vi "PH_TKTDS-30xx.Revision.vi"(0 "i ref in":refnum<vi>, 5 "error IO":errorcluster) -> (14 "i ref out":refnum<vi>, 19 "error out":errorcluster)   [LabVIEW 2014, in "PH_TKTDS-30xx.lvlib"]
doc: "If the connection is established, this VI queries the instrumnent driver revision, the instrument firmware revision, and errors which are written to own attributes."
uses:
  PH_TKTDS-30xx.lvlib
  instr.lib/TKDS3032-PHELIX/tktds3032-PHELIX - Driver np.lvlib
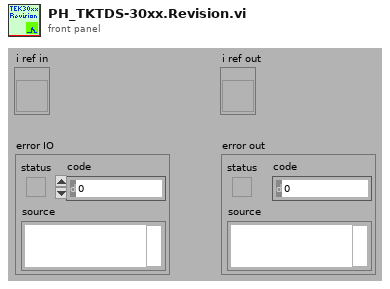
[diagram p1: front panel]
types:
  T1 = typedef "PH_TKTDS-30xx.lvlib/PH_TKTDS-30xx.i attribute.ctl" = cluster{"Default VISA Resource":string, "VISA Resource Name":refnum<visa-resource-name>, "Revision":cluster{"Instrument Driver":string, "Instrument Firmware":string}, "Selftest":cluster{"Result":u32, "Message":string}, "Channels":T2[], "Trigger Configuration":T3, "Acquisition Configuration":T4, "Fetched Waveforms":T5[], "GUI Refs":T6, "GUI Refs Channels":refnum<vi>[], "State":T7, "Error Message":string, "Allow Prdc Loop?":bool}
  T2 = typedef "PH_TKTDS-30xx.lvlib/PH_TKTDS-30xx.Channel Config.ctl" = cluster{"Channel Name":string, "Input Impedance":string, "Max Input Frequency":string, "Vertical Coupling":i32, "Channel Enabled":bool, "Probe Attenuation":dbl, "Vertical Range":dbl, "Vertical Offset":dbl}
  T3 = typedef "PH_TKTDS-30xx.lvlib/PH_TKTDS-30xx.Trigger Config.ctl" = cluster{"Source":string, "Slope":i32, "Level [V]":dbl}
  T4 = typedef "PH_TKTDS-30xx.lvlib/PH_TKTDS-30xx.Acquisition Config.ctl" = cluster{"Time base":dbl, "Record Length":u16, "Start Time":dbl, "Type":i32, "Continuous":bool}
  T5 = typedef "PH_TKTDS-30xx.lvlib/PH_TKTDS-30xx.fetched Waveform.ctl" = cluster{"Source":string, "Actual Points":u32, "Initial X":dbl, "X Increment":dbl, "Waveform Array":dbl[]}
  T6 = typedef "PH_TKTDS-30xx.lvlib/PH_TKTDS-30xx.GUI Refs.ctl" = cluster{"Trigger":refnum<vi>, "Acquisition":refnum<vi>, "Graph":refnum<vi>, "State":refnum<vi>, "Delete":refnum<vi>, "Channel to be positioned":refnum<vi>, "Postion":refnum<vi>, "Display Intensity":refnum<vi>, "VISA Resource":refnum<vi>}
  T7 = typedef "PH_StatusHandler.lvlib/PH_StatusHandler.Status.ctl" = i16
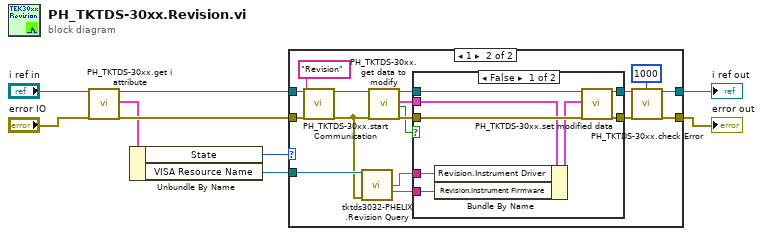
[diagram p0: block diagram]
diagram:
  n1 = call "PH_TKTDS-30xx.get i attribute.vi"("i ref in"="i ref in", "error in (no error)"="error IO") -> ("i ref out"=w3:refnum<vi>, "i attribute"=w5:T1, "error out"=w7:errorcluster)  [unwired: 15 in]
  n2 = Unbundle By Name(w5) -> ("State"=w9:T7, "VISA Resource Name"=w6:refnum<visa-resource-name>)
  n3 = case shown="1" w9 {
    tunnel: w3 -> [w11 w14]
    tunnel: w6 -> [_ w23]
    tunnel: w7 -> [w10 w22]
    tunnel: [w11 w18] -> w8
    tunnel: [w10 w16] -> w1
    frame Default {
    }
    frame 1 {
      n4 = call "PH_TKTDS-30xx.start Communication.vi"("i ref in"=w14, "Action"="Revision", "error in"=w22) -> ("i ref out"=w15:refnum<vi>, "error out"=w19:errorcluster)  [unwired: 15 in]
      n5 = call "tktds3032-PHELIX.Revision Query.vi"("VISA Resource Name"=w23, "error in (no error)"=w19) -> ("Instr Driver Revision"=w21:string, "Instr Firmware Revision"=w20:string)  [unwired: 10 in, 2 out]
      n6 = call "PH_TKTDS-30xx.get data to modify.vi"("i ref in"=w15, "error in (no error)"=w19) -> ("i ref out"=w26:refnum<vi>, "i attribute"=w24:T1, "timed out"=w25:bool, "error out"=w27:errorcluster)  [unwired: 14 in]
      n7 = case shown="False" w25 {
        tunnel: [w36 w37] -> w17
        tunnel: w27 -> [w35 w37]
        tunnel: w26 -> [w34 w38]
        tunnel: [w33 w38] -> w28
        tunnel: w24 -> [w32 _]
        tunnel: w21 -> [w30 _]
        tunnel: w20 -> [w29 _]
        frame False {
          n8 = Bundle By Name(cluster=w32, "Revision.Instrument Driver"=w30, "Revision.Instrument Firmware"=w29) -> (w31:T1)
          n9 = call "PH_TKTDS-30xx.set modified data.vi"("i ref in"=w34, "i attribute"=w31, "error in (no error)"=w35) -> ("i ref out"=w33:refnum<vi>, "error out"=w36:errorcluster)  [unwired: 15 in]
        }
        frame True {
        }
      }
      n10 = call "PH_TKTDS-30xx.check Error.vi"("i ref in"=w28, "Waiting Time [ms]"=u32 1000, "error in"=w17) -> ("i ref out"=w18:refnum<vi>, "error out"=w16:errorcluster)  [unwired: 15 in]
    }
  }
  "i ref out" <- w8
  "error out" <- w1
